vi "NCS_AmpPh_FilterOption.vi"(6 "Low-Pass Freq":dbl=200.0 format="%#_13g", 8 "IQ":cdb[](array[numeric]), 9 "data":cdb[][](array[numeric]), 10 "Sampling Rate":i32=500, 11 "Coerced Rx IQ Rate":dbl) -> (0 "Phase DownSampled":dbl[](array[numeric]), 1 "Amp DownSampled":dbl[](array[numeric]), 2 "Unfiltered Phase":dbl[](array[numeric]), 3 "Unfiltered Amplitude":dbl[](array[numeric]))   [LabVIEW 2016]
uses:
  <vilib>/Analysis/coordinate.llb/Wrap Angle (array).vi
  <vilib>/Analysis/3filter.llb/Butterworth Filter (DBL).vi
  <vilib>/Analysis/NI_AALBase.lvlib
  <vilib>/Analysis/NI_AALPro.lvlib
  <vilib>/Analysis/NI_AAL_Angle.lvlib
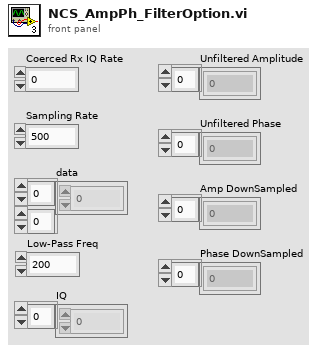
[diagram p1: front panel]
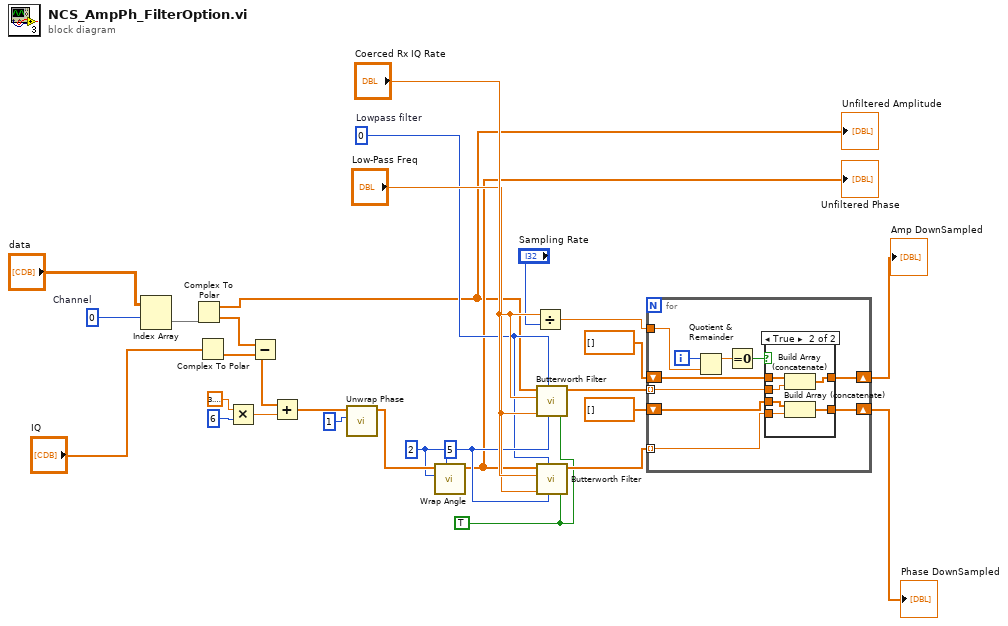
[diagram p0: block diagram]
diagram:
  w3 = 0  # Channel
  w22 = 5 ("order1")
  w17 = 2 ("y")
  w23 = TRUE
  w21 = 0  # Lowpass filter
  n1 = Index Array(array="data", index (row)=w3) -> (element=w1:cdb[])  [unwired: 1 in]
  n2 = Complex To Polar(r * e^(i*theta)=w1) -> (r=w7:dbl[], theta=w19:dbl[])
  "Unfiltered Amplitude" <- w7
  n3 = Complex To Polar(r * e^(i*theta)="IQ") -> (theta=w13:dbl[])  [unwired: 1 out]
  n4 = Multiply(x=3.141592653589793, y=6) -> (x*y=w12:dbl)
  n5 = Subtract(x=w19, y=w13) -> (x-y=w15:dbl[])
  n6 = Add(x=w15, y=w12) -> (x+y=w16:dbl[])
  n7 = call <vilib>:"Unwrap Phase.vi"("phase unit"=1 ("y"), "Phase"=w16) -> ("Unwrapped Phase"=w18:dbl[])  [unwired: 8 in, 1 out]
  n8 = call-poly <vilib>:"Wrap Angle.vi"("angle units"=w17, "angle range"=w17, "Angle In"=w18) -> ("Angle Out"=w20:dbl[])  [unwired: 7 in, 1 out]
  "Unfiltered Phase" <- w20
  n9 = Divide(x="Coerced Rx IQ Rate", y="Sampling Rate") -> (x/y=w6:dbl)
  n10 = call-poly <vilib>:"Butterworth Filter.vi"("init/cont (init:F)"=w23, "order"=w22, "filter type"=w21, "low cutoff freq: fl"="Low-Pass Freq", "sampling freq: fs"="Coerced Rx IQ Rate", "X"=w7) -> ("Filtered X"=w8:dbl[])  [unwired: 2 in, 1 out]
  n11 = call-poly <vilib>:"Butterworth Filter.vi"("init/cont (init:F)"=w23, "order"=w22, "filter type"=w21, "low cutoff freq: fl"="Low-Pass Freq", "sampling freq: fs"="Coerced Rx IQ Rate", "X"=w20) -> ("Filtered X"=w25:dbl[])  [unwired: 2 in, 1 out]
  n12 = for {
    tunnel: w8 -> [w39] mode=indexing
    shift-right: [w37] -> w28
    shift-left: dbl[] [] -> [w38]
    tunnel: w6 -> [w33]
    shift-right: [w31] -> w26
    shift-left: dbl[] [] -> [w32]
    tunnel: w25 -> [w30] mode=indexing
    i -> [w36]
    n13 = Quotient & Remainder(x=w36, y=w33) -> (x-y*floor(x/y)=w34:dbl)  [unwired: 1 out]
    n14 = Equal To 0?(x=w34) -> (x = 0?=w35:bool)
    n15 = case shown="True" w35 {
      tunnel: w39 -> [_ w47]
      tunnel: w38 -> [w41 w46]
      tunnel: [w41 w45] -> w37
      tunnel: w32 -> [w40 w44]
      tunnel: [w40 w43] -> w31
      tunnel: w30 -> [_ w42]
      frame False {
      }
      frame True {
        n16 = Build Array (concatenate)(w46, w47) -> (w45:dbl[])
        n17 = Build Array (concatenate)(w44, w42) -> (w43:dbl[])
      }
    }
  }
  "Amp DownSampled" <- w28
  "Phase DownSampled" <- w26
